vi "rollingArray_time (SubVI).vi"(10 "seconds since 1Jan1904":timestamp, 11 "Array in":timestamp[](array[timestamp])) -> (3 "Array out":timestamp[](array[timestamp]))   [LabVIEW 2014]
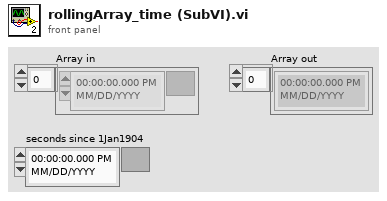
[diagram p1: front panel]
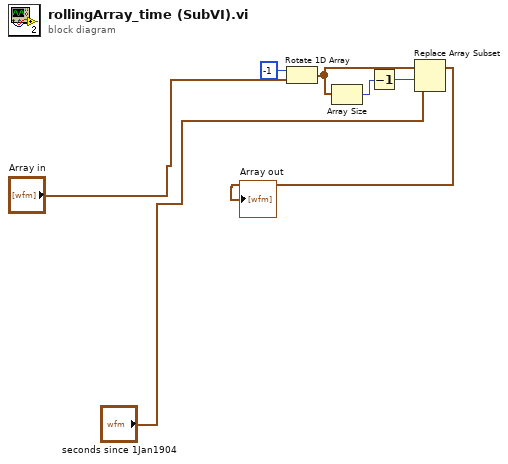
[diagram p0: block diagram]
diagram:
  n1 = Rotate 1D Array(1:"Array in", 2:-1 ("n")) -> (0:w2:timestamp[])
  n2 = Array Size(array=w2) -> (size(s)=w3:i32)
  n3 = Decrement(x=w3) -> (x-1=w4:i32)
  n4 = Replace Array Subset(array=w2, new element="seconds since 1Jan1904", index=w4) -> (→"Array out":timestamp[])
